vi "Write RFFE Adress.vi"(8 "error in (no error)":errorcluster, 10 "RFFE Address":u32=7 min=6 max=7 step=1, 11 "Toggle 6 in":refnum<class "Toggle 7.1.lvclass">) -> (0 "error out":errorcluster, 3 "Toggle 6 out":refnum<class "Toggle 7.1.lvclass">)   [LabVIEW 2020, in "Toggle 7.1.lvclass"]
uses:
  Toggle 7.1.lvclass
  Toggle 7.1.lvclass/Toggle 7.1.ctl
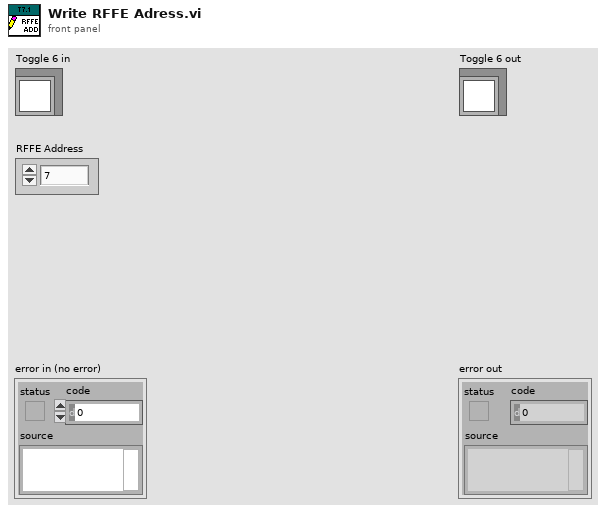
[diagram p1: front panel]
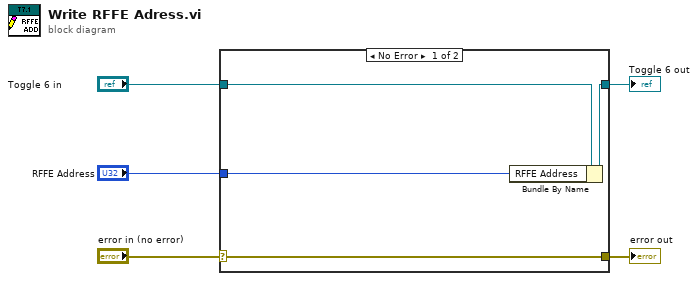
[diagram p0: block diagram]
diagram:
  n1 = case shown="No Error" "error in (no error)" {
    selector: "error in (no error)" -> [w9 w10]
    tunnel: [w9 w10] -> w4
    tunnel: [w7 w11] -> w2
    tunnel: "Toggle 6 in" -> [w8 w11]
    tunnel: "RFFE Address" -> [w6 _]
    frame No Error {
      n2 = Bundle By Name(cluster=w8, "RFFE Address"=w6) -> (w7:refnum<class "Toggle 7.1.lvclass">)
    }
    frame Error {
    }
  }
  "error out" <- w4
  "Toggle 6 out" <- w2
